vi "myRIO_BRig_RT_dataLC_ENL1_delayOpt_NS_l1.vi"() -> (2 "output_ENL1_delayOpt_NS_l1":i32)   [LabVIEW 2014]
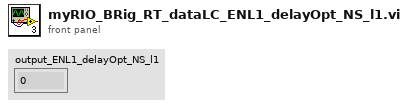
[diagram p1: front panel]
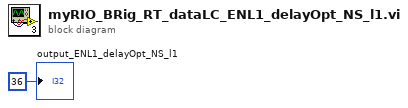
[diagram p0: block diagram]
diagram:
  "output_ENL1_delayOpt_NS_l1" <- 36 ("output_iBlock")
